vi "serial_write_and_read.vi"(0 "port name in":refnum<visa-resource-name>, 1 "reconnect?":bool, 2 "disconnect?":bool, 5 "write buffer":string, 7 "do writing?":bool, 9 "expecting response?":bool, 11 "error in":errorcluster, 12 "expected max length":u32=255, 13 "connection parameters":T1={"baud rate (9600)"=9600, "data bits (8)"=8, "stop bits (10: 1 bit)"=10, "parity (0:none)"=enum."None", "flow control (0:none)"=0, "timeout (10sec)"=10000, "Enable Termination\nChar (T)"=TRUE, "termination char\n(0xA = '\\n' = LF)\n(0xD = '\\r' = CF) "=13} {"flow control (0:none)" items=["None", "XON/XOFF", "RTS/CTS", "XON/XOFF & RTS/CTS", "DTR/DSR", "XON/XOFF & DTR/DSR"]; "stop bits (10: 1 bit)" items=["1.0"=10, "1.5"=15, "2.0"=20]}) -> (4 "port name out":refnum<visa-resource-name>, 6 "read buffer":string, 15 "error out":errorcluster)   [LabVIEW 2016]
uses:
  <vilib>/Instr/_visa.llb/VISA Flush IO Buffer Mask.ctl
  <vilib>/Instr/_visa.llb/VISA Configure Serial Port (Instr).vi
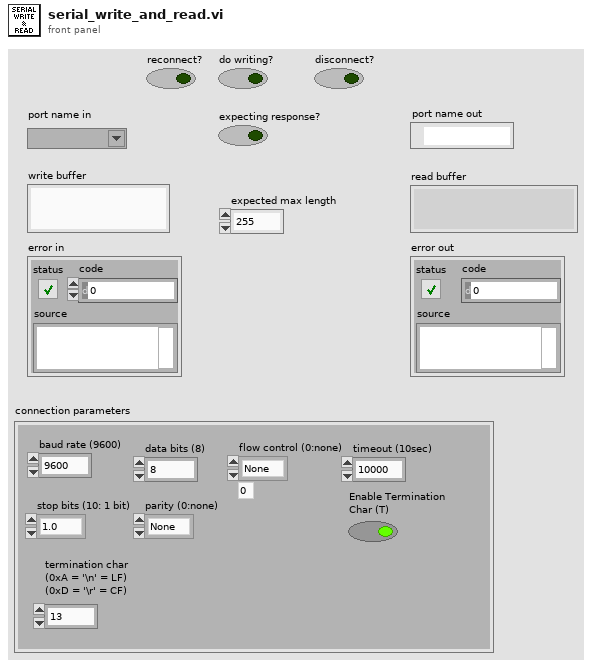
[diagram p1: front panel]
types:
  T1 = cluster{"baud rate (9600)":u32, "data bits (8)":u16, "stop bits (10: 1 bit)":u16, "parity (0:none)":enum16{"None", "Odd", "Even", "Mark", "Space"}, "flow control (0:none)":u16, "timeout (10sec)":u32, "Enable Termination\nChar (T)":bool, "termination char\n(0xA = '\\n' = LF)\n(0xD = '\\r' = CF) ":u8}
  T2 = typedef "VISA Flush IO Buffer Mask.ctl" = u16
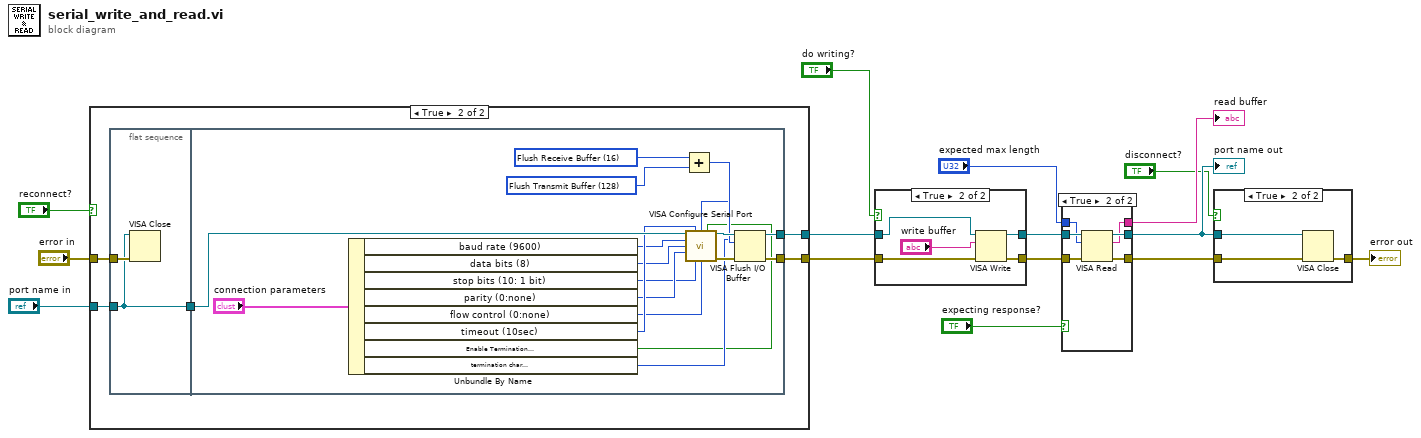
[diagram p0: block diagram]
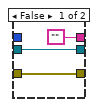
[diagram p5: hidden frame]
diagram:
  n1 = case shown="True" "reconnect?" {
    tunnel: "error in" -> [w16 w21]
    tunnel: [w16 w20] -> w12
    tunnel: [w17 w19] -> w11
    tunnel: "port name in" -> [w17 w18]
    frame False {
    }
    frame True {
      n2 = flat-sequence {
        tunnel: w21 -> [w24]
        tunnel: [w23] -> w22
        tunnel: w18 -> [w23]
        tunnel: w22 -> [w41]
        tunnel: [w39] -> w20
        tunnel: [w37] -> w19
        frame #0 {
          n3 = VISA Close(VISA resource name=w23, error in (no error)=w24) -> ()  [unwired: 1 out]
        }
        frame #1 {
          w35 = T2 128 items=["Flush Receive Buffer"=16, "Write Transmit Buffer to Device"=32, "Flush Receive Buffer (No I/O)"=64, "Flush Transmit Buffer"=128] ("Mask")
          w36 = T2 16 items=["Flush Receive Buffer"=16, "Write Transmit Buffer to Device"=32, "Flush Receive Buffer (No I/O)"=64, "Flush Transmit Buffer"=128] ("Mask")
          n4 = Unbundle By Name("connection parameters") -> ("baud rate (9600)"=w25:u32, "data bits (8)"=w26:u16, "stop bits (10: 1 bit)"=w27:u16, "parity (0:none)"=w28:enum16{"None", "Odd", "Even", "Mark", "Space"}, "flow control (0:none)"=w29:u16, "timeout (10sec)"=w30:u32, "Enable Termination\nChar (T)"=w31:bool, "termination char\n(0xA = '\\n' = LF)\n(0xD = '\\r' = CF)"=w32:u8)
          n5 = Add(x=w36, y=w35) -> (x+y=w34:T2)
          n6 = call-poly "VISA Configure Serial Port"("VISA resource name"=w41, "timeout (10sec)"=w30, "termination char\n(0xA = '\\n' = LF)"=w32, "Enable Termination\nChar (T)"=w31, "baud rate (9600)"=w25, "data bits (8)"=w26, "parity (0:none)"=w28, "stop bits (10: 1 bit)"=w27, "flow control (0:none)"=w29) -> ("VISA resource name out"=w38:refnum<visa-resource-name>, "error out"=w40:errorcluster)  [unwired: 5 in]
          n7 = VISA Flush I/O Buffer(VISA resource name=w38, mask (16)=w34, error in (no error)=w40) -> (VISA resource name out=w37:refnum<visa-resource-name>, error out=w39:errorcluster)
        }
      }
    }
  }
  n8 = case shown="True" "do writing?" {
    tunnel: [w42 w48] -> w14
    tunnel: [w43 w47] -> w13
    tunnel: w12 -> [w42 w46]
    tunnel: w11 -> [w43 w45]
    frame False {
    }
    frame True {
      n9 = VISA Write(VISA resource name=w45, write buffer="write buffer", error in (no error)=w46) -> (VISA resource name out=w47:refnum<visa-resource-name>, error out=w48:errorcluster)  [unwired: 1 out]
    }
  }
  n10 = case shown="True" "expecting response?" {
    tunnel: w14 -> [w50 w57]
    tunnel: w13 -> [w51 w56]
    tunnel: [w50 w55] -> w7
    tunnel: [w51 w54] -> w6
    tunnel: ["" w53] -> w9
    tunnel: "expected max length" -> [_ w52]
    frame False {
    }
    frame True {
      n11 = VISA Read(VISA resource name=w56, byte count=w52, error in (no error)=w57) -> (VISA resource name out=w54:refnum<visa-resource-name>, read buffer=w53:string, error out=w55:errorcluster)  [unwired: 1 out]
    }
  }
  "read buffer" <- w9
  "port name out" <- w6
  n12 = case shown="True" "disconnect?" {
    tunnel: w7 -> [w58 w61]
    tunnel: w6 -> [_ w60]
    tunnel: [w58 w59] -> w1
    frame False {
    }
    frame True {
      n13 = VISA Close(VISA resource name=w60, error in (no error)=w61) -> (error out=w59:errorcluster)
    }
  }
  "error out" <- w1
